vi "subscriber.vi"() -> ()   [LabVIEW 2015]
doc: "Sample subscriber. Subscribes to the topic chatter"
uses:
  <userlib>/ROS for LabVIEW Software/ROS/Code/Console/Servers/ServerSubs/TopicDef.ctl
  <userlib>/ROS for LabVIEW Software/ROS/Code/SubVIs/_ROSDirection.ctl
  <userlib>/ROS for LabVIEW Software/ROS/MessageParsing/std_msgs/subs/parse_string_scalar.vi
panel:
  out "Cluster":cluster{"x":dbl, "y":dbl, "z":dbl}
  in  "stop":bool
  out "error out":errorcluster
  out "I heard:":string
  # "Instructions:\n1. Run Publisher example\n2. Run Subscriber eample"
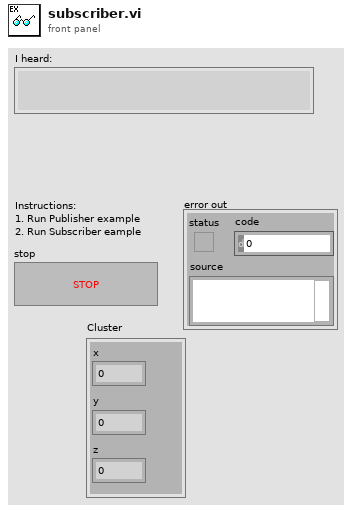
[diagram p1: front panel]
types:
  T1 = typedef "TopicDef.ctl" = cluster{"Topic":string, "Type":string, "Action":T2, "Update (ms)":u16, "queue size":u16}
  T2 = typedef "_ROSDirection.ctl" = enum16{"Node", "Publisher", "Subscriber", "ServiceClient", "ServiceProvider"}
  T3 = typedef "_ROSControl.ctl" = cluster{"topic port":u16, "Node":string, "topic":string, "type":string, "node port":u16, "error ":errorcluster, "Direction":T2, "Update (ms)":u16, "FIFO size":u16}
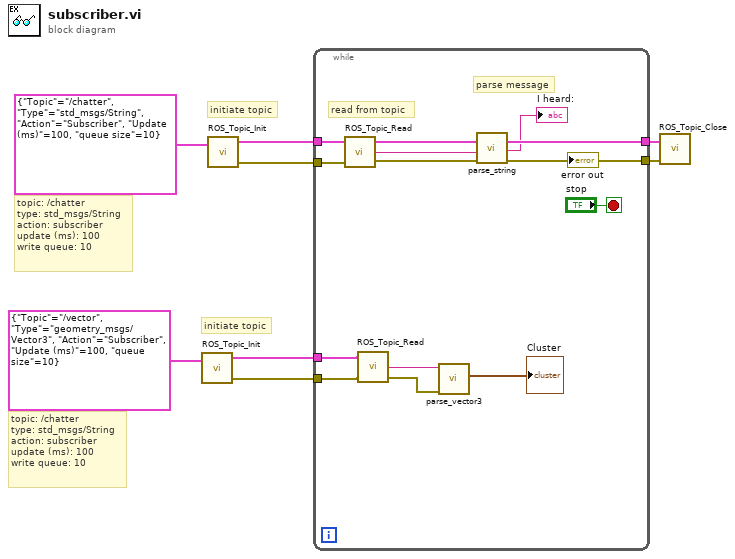
[diagram p0: block diagram]
diagram:
  # "initiate topic"
  # "topic: /chatter\ntype: std_msgs/String\naction: subscriber\nupdate (ms): 100\nwrite queue: 10"
  # "initiate topic"
  # "topic: /chatter\ntype: std_msgs/String\naction: subscriber\nupdate (ms): 100\nwrite queue: 10"
  n1 = call <userlib>:"ROS_Topic_Init.vi"("Definitions"=T1 {"Topic"="/vector", "Type"="geometry_msgs/Vector3", "Action"=enum."Subscriber", "Update (ms)"=100, "queue size"=10}) -> ("ROS out"=w2:T3, "error out"=w1:errorcluster)  [unwired: 2 in]
  n2 = call <userlib>:"ROS_Topic_Init.vi"("Definitions"=T1 {"Topic"="/chatter", "Type"="std_msgs/String", "Action"=enum."Subscriber", "Update (ms)"=100, "queue size"=10}) -> ("ROS out"=w7:T3, "error out"=w6:errorcluster)  [unwired: 2 in]
  n3 = while {
    tunnel: w7 -> [w21]
    tunnel: w6 -> [w20]
    tunnel: [w18] -> w5
    tunnel: [w9] -> w4
    tunnel: w2 -> [w14]
    tunnel: w1 -> [w13]
    stop <- "stop" stop-if-true
    # "parse message"
    # "read from topic"
    n4 = call <userlib>:"ROS_Topic_Read.vi"("error in (no error)"=w20, "ROS in"=w21) -> ("error out"=w15:errorcluster, "Reply"=w17:string, "ROS out"=w18:T3)  [unwired: 1 in]
    n5 = call <userlib>:"ROS_Topic_Read.vi"("error in (no error)"=w13, "ROS in"=w14) -> ("error out"=w10:errorcluster, "Reply"=w12:string)  [unwired: 1 in, 1 out]
    n6 = call <vilib>:"parse_vector3.vi"("error in"=w10, "msg in"=w12) -> ("Vector3"=→"Cluster":cluster{"x":dbl, "y":dbl, "z":dbl})  [unwired: 3 in, 2 out]
    n7 = call-poly <userlib>:"parse_string.vi"("error in"=w15, "msg in"=w17) -> ("error out"=w9:errorcluster, "string"=→"I heard:":string)  [unwired: 3 in, 1 out]
    "error out" <- w9
  }
  n8 = call <userlib>:"ROS_Topic_Close.vi"("error in"=w4, "ROS in"=w5) -> ()  [unwired: 2 in, 1 out]
